vi "Tricon Wait until Finished.vi"(6 "Timeout(s)":i16=10, 7 "Pump Address":T1, 8 "error out":errorcluster, 11 "VISA resource name in":refnum<visa-resource-name>) -> (0 "error out":errorcluster, 1 "Cancelled":bool, 2 "Error Code":string, 3 "VISA resource name out":refnum<visa-resource-name>)   [LabVIEW 2018]
uses:
  Pump Address.ctl
  Main/Main Globals.vi
panel:
  out "Elapsed Time":bool
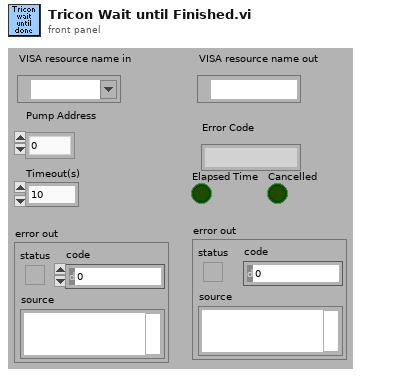
[diagram p1: front panel]
types:
  T1 = typedef "Pump Address.ctl" = enum16{"0", "1", "2", "3", "4", "5", "6", "7"}
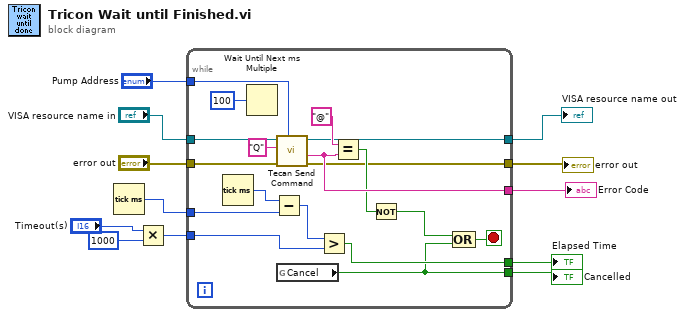
[diagram p0: block diagram]
diagram:
  n1 = Tick Count (ms)() -> (millisecond timer value=w6:u32)
  n2 = Multiply(x="Timeout(s)", y=i16 1000) -> (x*y=w5:i16)
  n3 = while {
    tunnel: "VISA resource name in" -> [w30]
    tunnel: "error out" -> [w20]
    tunnel: [w14] -> w10
    tunnel: [w27] -> w9
    tunnel: w6 -> [w25]
    tunnel: w5 -> [w22]
    tunnel: "Pump Address" -> [w21]
    tunnel: [w15] -> w3
    tunnel: [w16] -> w2
    tunnel: [w13] -> w1
    stop <- w24 stop-if-true
    n4 = Tick Count (ms)() -> (millisecond timer value=w26:u32)
    n5 = Wait Until Next ms Multiple(millisecond multiple=u32 100 ("Delay (ms)")) -> ()  [unwired: 1 out]
    n6 = Subtract(x=w26, y=w25) -> (x-y=w23:u32)
    n7 = call "Tecan Send Command.vi"("Address"=w21, "error in (no error)"=w20, "Command"="Q", "VISA resource name in"=w30) -> ("error out"=w14:errorcluster, "Status Code"=w27:string, "VISA resource name out"=w15:refnum<visa-resource-name>)  [unwired: 3 in, 2 out]
    n8 = global read "Main Globals.vi" "Cancel"() -> (w13:bool)
    n9 = Greater?(x=w23, y=w22) -> (0:w16:bool)
    n10 = Equal?(x="@", y=w27) -> (x = y?=w18:bool)
    n11 = Not(x=w18) -> (.not. x?=w17:bool)
    n12 = Compound Arithmetic op=OR(w17, w13) -> (w24:bool)
  }
  "VISA resource name out" <- w3
  "error out" <- w10
  "Error Code" <- w9
  "Elapsed Time" <- w2
  "Cancelled" <- w1
